vi "Test Shutdown Procedure.vi"(8 "error in (no error)":errorcluster) -> (0 "error out":errorcluster)   [LabVIEW 2016, in "Hall Effect Library.lvlib"]
uses:
  Hall Effect Library.lvlib
  Public/Controls/Switches.ctl
  Public/Controls/Voltmeters.ctl
  Global Variables/Instrument Locations.vi
  Global Variables/Instruments.vi
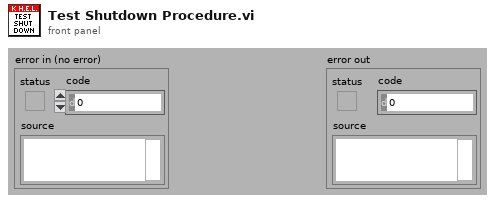
[diagram p1: front panel]
types:
  T1 = typedef "Hall Effect Library.lvlib/Voltmeters.ctl" = enum16{"2000", "2182A", "3706A"}
  T2 = typedef "Hall Effect Library.lvlib/Switches.ctl" = enum16{"3706A"}
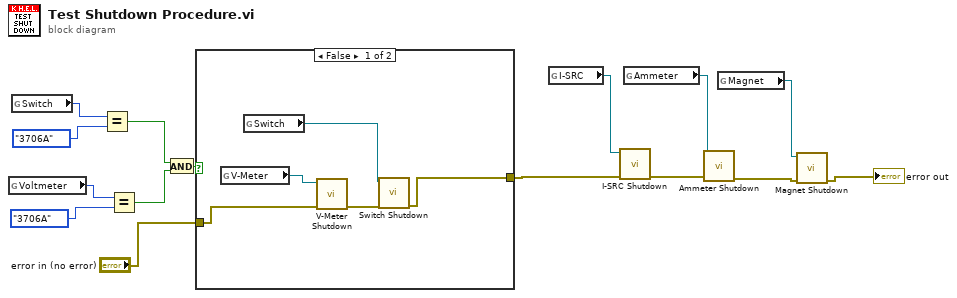
[diagram p0: block diagram]
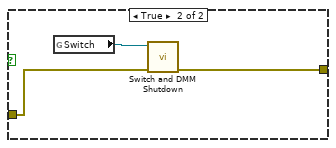
[diagram p2: hidden frame]
diagram:
  n1 = global read "Instruments.vi" "Voltmeter"() -> (w13:T1)
  n2 = global read "Instruments.vi" "Switch"() -> (w15:T2)
  n3 = Equal?(x=w15, y=Switches."3706A" ("Switch")) -> (x = y?=w11:bool)
  n4 = Equal?(x=w13, y=Voltmeters."3706A" ("Voltmeter")) -> (x = y?=w10:bool)
  n5 = And(x=w11, y=w10) -> (x .and. y?=w9:bool)
  n6 = case shown="False" w9 {
    tunnel: "error in (no error)" -> [w18 w22]
    tunnel: [w16 w21] -> w6
    frame False {
      n7 = global read "Instrument Locations.vi" "V-Meter"() -> (w20:refnum<visa-resource-name>)
      n8 = global read "Instrument Locations.vi" "Switch"() -> (w19:refnum<visa-resource-name>)
      n9 = call "V-Meter Shutdown.vi"("error in (no error)"=w18, "VISA resource name in"=w20) -> ("error out"=w17:errorcluster)  [unwired: 9 out]
      n10 = call "Switch Shutdown.vi"("error in (no error)"=w17, "VISA resource name in"=w19) -> ("error out"=w16:errorcluster)  [unwired: 9 out]
    }
    frame True {
      n11 = global read "Instrument Locations.vi" "Switch"() -> (w23:refnum<visa-resource-name>)
      n12 = call "Switch and DMM Shutdown.vi"("error in (no error)"=w22, "VISA resource name"=w23) -> ("error out"=w21:errorcluster)  [unwired: 8 in, 1 out]
    }
  }
  n13 = global read "Instrument Locations.vi" "I-SRC"() -> (w7:refnum<visa-resource-name>)
  n14 = call "I-SRC Shutdown.vi"("error in (no error)"=w6, "VISA resource name in"=w7) -> ("error out"=w5:errorcluster)  [unwired: 9 out]
  n15 = global read "Instrument Locations.vi" "Ammeter"() -> (w4:refnum<visa-resource-name>)
  n16 = call "Ammeter Shutdown.vi"("error in (no error)"=w5, "VISA resource name in"=w4) -> ("error out"=w2:errorcluster)  [unwired: 9 out]
  n17 = global read "Instrument Locations.vi" "Magnet"() -> (w3:refnum<visa-resource-name>)
  n18 = call "Magnet Shutdown.vi"("error in (no error)"=w2, "VISA resource name in"=w3) -> ("error out"=→"error out":errorcluster)  [unwired: 9 out]
